vi "grabimg.vi"(7 "array in":u16[][](array[numeric]), 8 "error in":errorcluster, 11 "Hin":u64) -> (0 "error out":errorcluster, 2 "imgdata":i32[][](array[numeric]), 3 "Hout":u64)   [LabVIEW 2020]
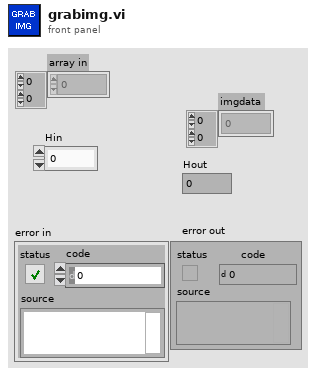
[diagram p1: front panel]
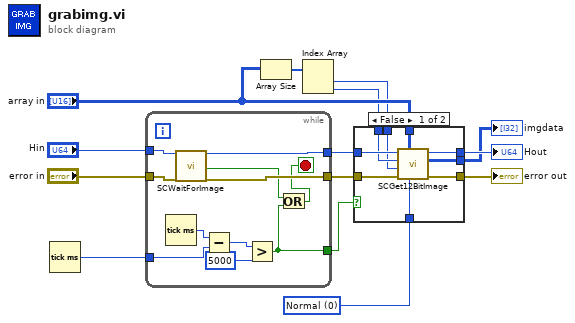
[diagram p0: block diagram]
diagram:
  w10 = 0 items=["Normal", "Upside down"] ("mode")
  n1 = Tick Count (ms)() -> (millisecond timer value=w2:u32)
  n2 = while {
    tunnel: [w25] -> w8
    tunnel: [w24] -> w9
    tunnel: "Hin" -> [w23]
    tunnel: "error in" -> [w22]
    tunnel: w2 -> [w20]
    tunnel: [w15] -> w1
    stop <- w16 stop-if-true
    n3 = Tick Count (ms)() -> (millisecond timer value=w21:u32)
    n4 = call "SCWaitForImage.vi"("Handle"=w23, "error in (no error)"=w22) -> ("Hout"=w24:u64, "Image Valid"=w17:bool, "error out"=w25:errorcluster)  [unwired: 15 in]
    n5 = Subtract(x=w21, y=w20) -> (x-y=w19:u32)
    n6 = Greater?(x=w19, y=u32 5000) -> (0:w15:bool)
    n7 = Or(x=w17, y=w15) -> (x .or. y?=w16:bool)
  }
  n8 = Array Size(array="array in") -> (size(s)=w5:i32[])
  n9 = Index Array(array=w5) -> (element #1=w3:i32, element #2=w4:i32)  [unwired: 2 in]
  n10 = case shown="False" w1 {
    tunnel: [w34 w35] -> w12
    tunnel: [w33 w36] -> w11
    tunnel: w10 -> [w32 _]
    tunnel: w9 -> [w31 w36]
    tunnel: w8 -> [w30 w35]
    tunnel: [w29 w37] -> w7
    tunnel: "array in" -> [w28 w37]
    tunnel: w4 -> [w27 _]
    tunnel: w3 -> [w26 _]
    frame False {
      n11 = call "SCGet12BitImage.vi"("mode"=w32, "Input array"=w28, "error in (no error)"=w30, "Vertical size"=w26, "Horizontal size"=w27, "Handle"=w31) -> ("error out"=w34:errorcluster, "imgdata"=w29:u16[][], "Hout"=w33:u64)  [unwired: 1 in]
    }
    frame True {
    }
  }
  "Hout" <- w11
  "imgdata" <- w7
  "error out" <- w12
